vi "CreateFolder.vi"(8 "error in (no error)":errorcluster, 10 "name":string, 11 "base path":path) -> (0 "error out":errorcluster, 3 "path out":path)   [LabVIEW 2018]
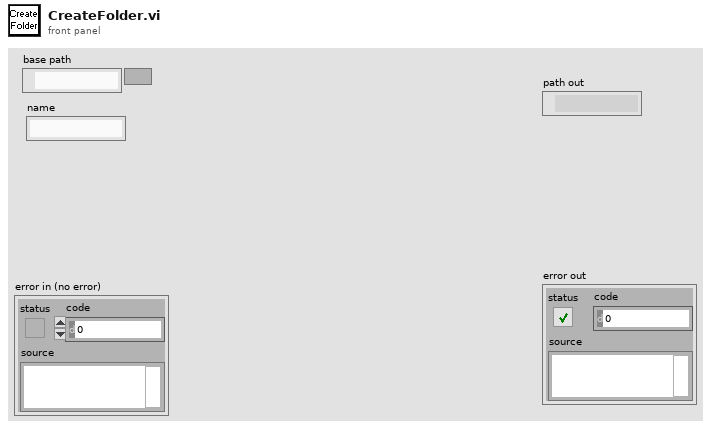
[diagram p1: front panel]
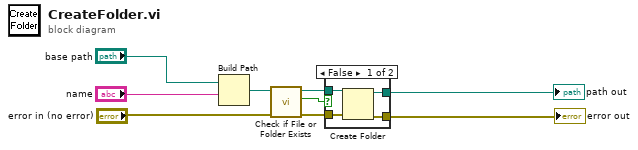
[diagram p0: block diagram]
diagram:
  n1 = Build Path(base path="base path", name or relative path="name") -> (appended path=w9:path)
  n2 = call <vilib>:"Check if File or Folder Exists.vi"("error in (no error)"="error in (no error)", "path"=w9) -> ("error out"=w7:errorcluster, "file or folder exists?"=w8:bool, "dup path"=w6:path)  [unwired: 7 in]
  n3 = case shown="False" w8 {
    tunnel: w7 -> [w13 w14]
    tunnel: [w12 w14] -> w4
    tunnel: [w11 w15] -> w3
    tunnel: w6 -> [w10 w15]
    frame False {
      n4 = Create Folder(path (use dialog)=w10, error in=w13) -> (created path=w11:path, error out=w12:errorcluster)  [unwired: 1 in, 1 out]
    }
    frame True {
    }
  }
  "error out" <- w4
  "path out" <- w3
